vi "Printer Error Handler.vi"(8 "error in (no error)":errorcluster, 10 "Queue Data":string, 11 "State In":T1) -> (0 "error out":errorcluster, 3 "Next State":T1)   [LabVIEW 2016]
doc: "Use this template to build a VI to use as a subVI."
uses:
  Print Processing States.ctl
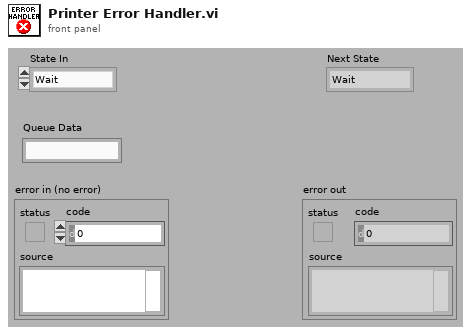
[diagram p1: front panel]
types:
  T1 = typedef "Print Processing States.ctl" = enum16{"Wait", "Initialize Setup", "Setup", "Initialize Print", "Print", "Shutdown"}
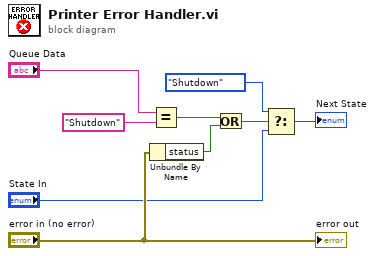
[diagram p0: block diagram]
diagram:
  n1 = Unbundle By Name("error in (no error)") -> ("status"=w6:bool)
  n2 = Equal?(x="Queue Data", y="Shutdown") -> (x = y?=w5:bool)
  n3 = Or(x=w5, y=w6) -> (x .or. y?=w4:bool)
  n4 = Select(t=Print_Processing_States."Shutdown", s=w4, f="State In") -> (s? t:f=→"Next State":T1)
  "error out" <- "error in (no error)"
